vi "Shared variable.vi"() -> ()   [LabVIEW 2017]
uses:
  <vilib>/Analysis/Matrix/Datatypes/RealMatrix.ctl
  <vilib>/Analysis/Matrix/Numeric/Multiply/Multiply - RM,RM.vi
  <vilib>/Analysis/Matrix/NI_Matrix.lvlib
panel:
  out "A + B":T1
  in  "Real Matrix 2":T1
  in  "Real Matrix":T1
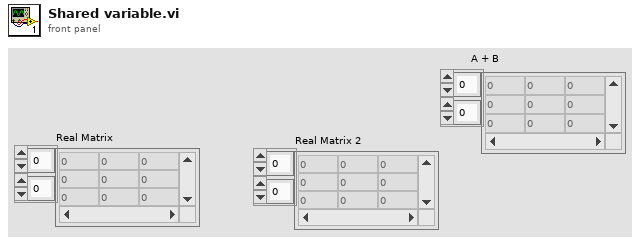
[diagram p1: front panel]
types:
  T1 = typedef "NI_Matrix.lvlib/RealMatrix.ctl" = dbl[][]
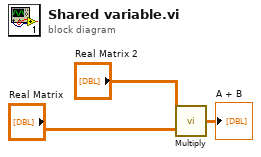
[diagram p0: block diagram]
diagram:
  n1 = call-poly <vilib>:"Multiply.vi"("Real Matrix B"="Real Matrix", "Real Matrix A"="Real Matrix 2") -> ("A * B"=→"A + B":T1)
